vi "模2加.vi"(1 "b":u32, 2 "a":u32) -> (0 "c":u32)   [LabVIEW 2013]
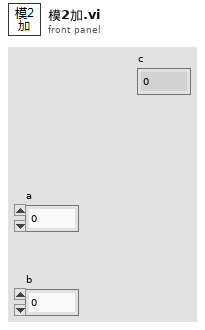
[diagram p1: front panel]
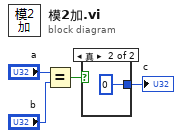
[diagram p0: block diagram]
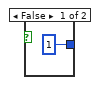
[diagram p2: hidden frame]
diagram:
  n1 = Equal?(x="a", y="b") -> (x = y?=w2:bool)
  n2 = case shown="真" w2 {
    tunnel: [1 0] -> w1
    frame False {
    }
    frame True {
    }
  }
  "c" <- w1
